vi "ERIO RT Save Signal As TDMS.vi"(8 "error in (no error)":errorcluster, 9 "TDMS File Folder In":path, 11 "Signal Capture":waveform(dbl)) -> (0 "error out":errorcluster, 1 "TDMS File Path Out":path)   [LabVIEW 2017]
doc: "Will input the signal waveform and save as a TDMS file. \n\nJames Tillett P.E.\nEndeavor Engineering Inc.\nwww.endeavoreng.com"
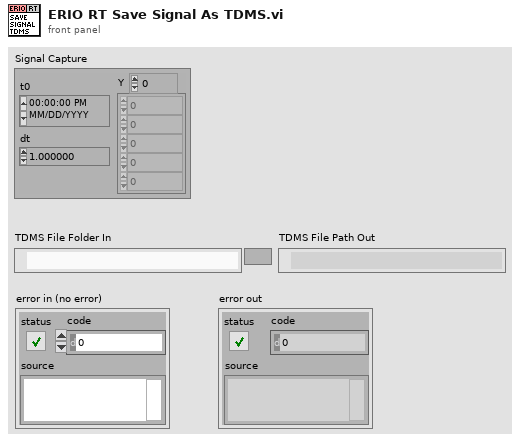
[diagram p1: front panel]
types:
  T1 = enum16{"open", "open or create", "create or replace", "create", "open (read-only)"}
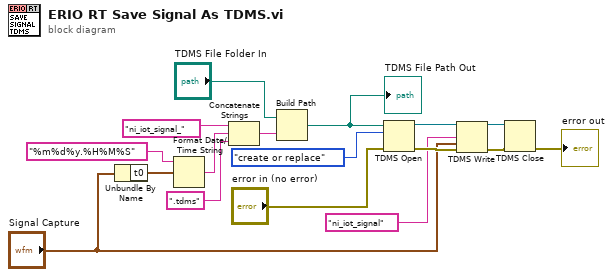
[diagram p0: block diagram]
diagram:
  n1 = Unbundle By Name("Signal Capture") -> ("t0"=w8:timestamp)
  n2 = Format Date/Time String(time format string (%c)="%m%d%y.%H%M%S", seconds (now)=w8) -> (date/time string=w5:string)  [unwired: 1 in]
  n3 = Concatenate Strings("ni_iot_signal_", w5, ".tdms") -> (w3:string)
  n4 = Build Path(base path="TDMS File Folder In", name or relative path=w3) -> (appended path=w1:path)
  "TDMS File Path Out" <- w1
  n5 = TDMS Open(8:"error in (no error)", 10:T1."create or replace" ("operation (0:open)"), 11:w1) -> (0:w14:errorcluster, 3:w15:refnum<k34>)  [unwired: 4 in]
  n6 = TDMS Write(0:w15, 7:"ni_iot_signal" ("channel name(s) in (Untitled)"), 9:"Signal Capture", 11:w14) -> (4:w12:refnum<k34>, 15:w11:errorcluster)  [unwired: 2 in, 2 out]
  n7 = TDMS Close(8:w11, 11:w12) -> (0:→"error out":errorcluster)  [unwired: 1 out]
